vi "Convert Controls to Arrays.vi"(4 "Sort Order":i32, 6 "Sort Column":i32, 8 "Top-Level Only?":bool, 9 "ConPane Only?":bool, 11 "Controls Data":refnum<class "Control.lvclass">[](array[class])) -> (3 "Control Array":string[][](array[string]))   [LabVIEW 2020, in "VI Properties Editor.lvlib"]
doc: "Converts <B>Controls Data</B> to arrays to be displayed to the user."
uses:
  VI Properties Editor.lvlib
  Classes/Control/Control.lvclass
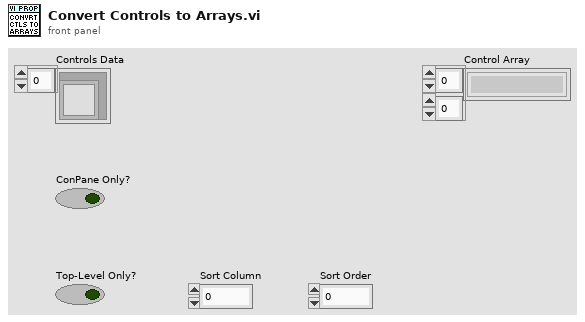
[diagram p1: front panel]
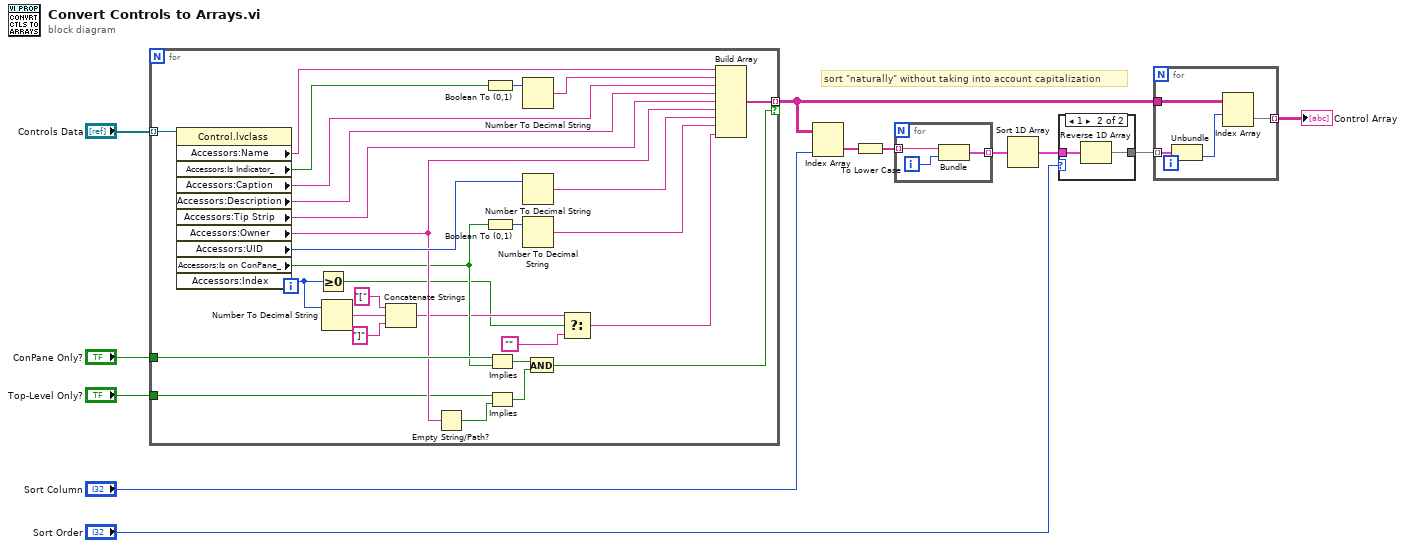
[diagram p0: block diagram]
diagram:
  # "sort \"naturally\" without taking into account capitalization"
  n1 = for {
    tunnel: [w38] -> w3 mode=indexing if=w22
    tunnel: "Controls Data" -> [w34] mode=indexing
    tunnel: "ConPane Only?" -> [w37]
    tunnel: "Top-Level Only?" -> [w25]
    n2 = property class="Control.lvclass"(reference=w34) -> ("Accessors:Name"=w33:string, "Accessors:Is Indicator_"=w32:bool, "Accessors:Caption"=w31:string, "Accessors:Description"=w30:string, "Accessors:Tip Strip"=w29:string, "Accessors:Owner"=w26:string, "Accessors:UID"=w28:i32, "Accessors:Is on ConPane_"=w18:bool, "Accessors:Index"=w14:i32)  [unwired: 1 in, 2 out]
    n3 = Greater Or Equal To 0?(x=w14) -> (x >= 0?=w13:bool)
    n4 = Number To Decimal String(number=w14) -> (decimal integer string=w21:string)  [unwired: 1 in]
    n5 = Concatenate Strings("[", w21, "]") -> (w17:string)
    n6 = Empty String/Path?(string/path=w26) -> (empty?=w23:bool)
    n7 = Boolean To (0,1)(Boolean=w32) -> (0, 1=w41:i16)
    n8 = Boolean To (0,1)(Boolean=w18) -> (0, 1=w36:i16)
    n9 = Implies(1:w18, 2:w37) -> (0:w27:bool)
    n10 = Implies(1:w23, 2:w25) -> (0:w24:bool)
    n11 = Number To Decimal String(number=w41) -> (decimal integer string=w40:string)  [unwired: 1 in]
    n12 = Number To Decimal String(number=w28) -> (decimal integer string=w39:string)  [unwired: 1 in]
    n13 = Number To Decimal String(number=w36) -> (decimal integer string=w35:string)  [unwired: 1 in]
    n14 = And(x=w27, y=w24) -> (x .and. y?=w22:bool)
    n15 = Select(t=w17, s=w13, f="") -> (s? t:f=w15:string)
    n16 = Build Array(w33, w40, w31, w30, w29, w26, w39, w35, w15) -> (w38:string[])
  }
  n17 = Index Array(array=w3, index (col)="Sort Column") -> (element=w7:string[])  [unwired: 1 in]
  n18 = To Lower Case(string=w7) -> (all lower case string=w6:string[])
  n19 = for {
    tunnel: w6 -> [w44] mode=indexing
    tunnel: [w42] -> w5 mode=indexing
    i -> [w43]
    n20 = Bundle("Accessors:Owner"=w44, w43) -> (w42:cluster{"Accessors:Owner":string, i32})  [unwired: 1 in]
  }
  n21 = Sort 1D Array(array=w5) -> (sorted array=w4:cluster{"Accessors:Owner":string, i32}[])
  n22 = case shown="1" "Sort Order" {
    tunnel: w4 -> [w45 w47]
    tunnel: [w45 w46] -> w2
    frame 0, Default {
    }
    frame 1 {
      n23 = Reverse 1D Array(array=w47) -> (reversed array=w46:cluster{"Accessors:Owner":string, i32}[])
    }
  }
  n24 = for {
    tunnel: w3 -> [w50]
    tunnel: w2 -> [w51] mode=indexing
    tunnel: [w48] -> w1 mode=indexing
    n25 = Unbundle(w51) -> (w49:i32)  [unwired: 1 out]
    n26 = Index Array(array=w50, index (row)=w49) -> (element=w48:string[])  [unwired: 1 in]
  }
  "Control Array" <- w1
